vi "mxwScript_API_XMLWireToTerminalByTermplateID.vi"(8 "error in (no error)":errorcluster, 10 "templateID":string, 11 "connector name":string) -> (0 "error out":errorcluster, 3 "encoded connector name":string)   [LabVIEW 2020]
doc: "Create encoded control name for connecting to a terminal on a generic node instead of to a control terminal. Terminal is specified by name. If multiple terminals with the same name exist, the first one is used.\n\nThis encoding works for both connected to and connected from terminals."
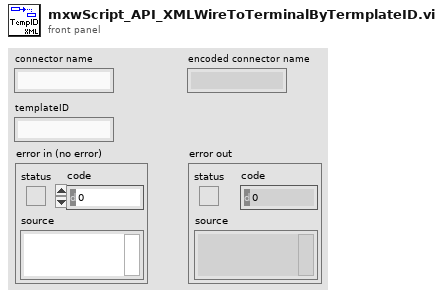
[diagram p1: front panel]
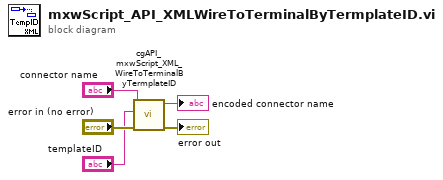
[diagram p0: block diagram]
diagram:
  n1 = call "cgAPI_mxwScript_XML_WireToTerminalByTermplateID.vi"("error in (no error)"="error in (no error)", "templateID"="templateID", "connector name"="connector name") -> ("error out"=→"error out":errorcluster, "encoded connector name"=→"encoded connector name":string)  [unwired: 7 out]
